vi "Check Channels Name.vi"(0 "data in":T1) -> (4 "data out":T1)   [LabVIEW 2019, in "GUI Sensor Lib.lvclass"]
uses:
  GUI Sensor Lib.lvclass
  TypeDef/CalibrationData.ctl
  TypeDef/GUI Setting Channel.ctl
  TypeDef/GUI AI Ranges.ctl
  TypeDef/Scale Data.ctl
panel:
  # "SCALED"
  # "SCALED"
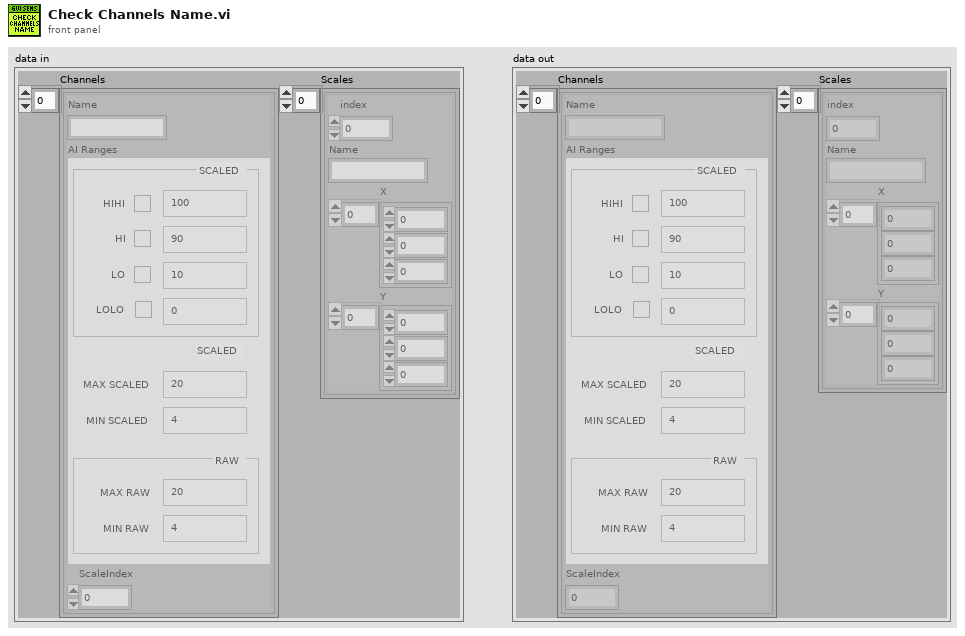
[diagram p1: front panel]
types:
  T1 = typedef "CalibrationData.ctl" = cluster{"Channels":T2[], "Scales":T4[]}
  T2 = typedef "GUI Setting Channel.ctl" = cluster{"Name":string, "AI Ranges":T3, "ScaleIndex":u32}
  T3 = typedef "GUI AI Ranges.ctl" = cluster{"HI":bool, "HIHI":bool, "LO":bool, "LOLO":bool, "HIHI VAL":dbl, "HI VAL":dbl, "LO VAL":dbl, "LOLO VAL":dbl, "MAX RAW":dbl, "MIN RAW":dbl, "MAX SCALED":dbl, "MIN SCALED":dbl}
  T4 = typedef "Scale Data.ctl" = cluster{"index":i32, "Name":string, "X":dbl[], "Y":dbl[]}
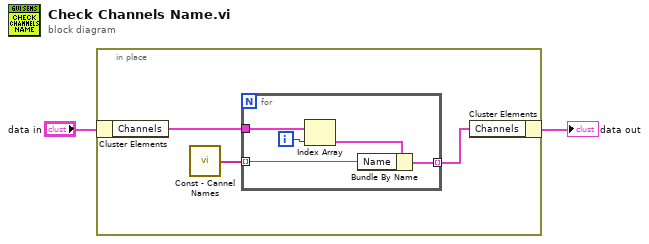
[diagram p0: block diagram]
diagram:
  n1 = in-place {
    n2 = in-place-cluster #1("data in") -> ("Channels"=w4:T2[])
    n3 = call "Const - Cannel Names.vi"() -> ("Channel Name"=w5:string[])
    n4 = for {
      tunnel: w5 -> [w7] mode=indexing
      tunnel: w4 -> [w10]
      tunnel: [w6] -> w3 mode=indexing
      i -> [w9]
      n5 = Index Array(array=w10, index=w9) -> (element=w8:T2)
      n6 = Bundle By Name(cluster=w8, "Name"=w7) -> (w6:T2)
    }
    n7 = in-place-cluster #1("Channels"=w3) -> (→"data out":T1)
  }
